vi "SetFieldTCRunner.vi"() -> ()   [LabVIEW 2019]
uses:
  Components/B_Globals.vi
  Components/DeltaRamp_globals.vi
  Components/Global 2.vi
panel:
  out "Numeric":i32
  in  "Settle [s]":dbl=60.0
  in  "Base Name":string="RT_100uA_dir=vir"
  in  "Start":bool
  in  "Directory":path=path "C:/User Data/gy251/2021628 AEN019D"
  in  "T_high":dbl=4.5
  in  "T_low":dbl=2.5
  in  "T_rate":dbl=0.1
  in  "B _rate":dbl=0.2
  in  "Set Fields":dbl[](array[numeric])=[0.0, 0.1, 0.2, 0.3, 0.4, 0.5, 0.6, 0.7, 0.8, 0.9, 1.0, 1.2, 1.4, 1.6, 1.8, 2.0]
  out "Action":string="Starting Measurement"
  out "Output File":path=path "RT_100uA_dir=vir_set=0p00T"
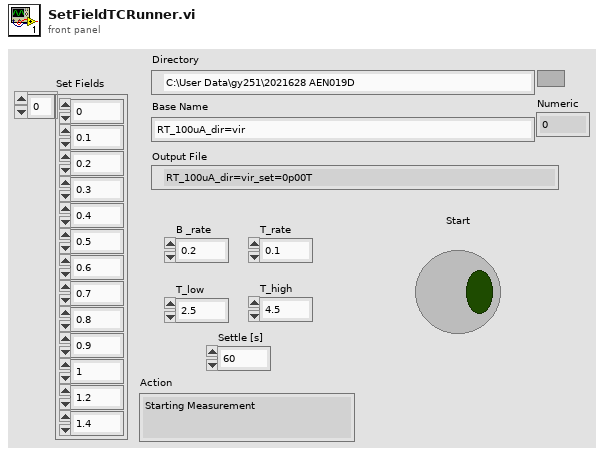
[diagram p1: front panel]
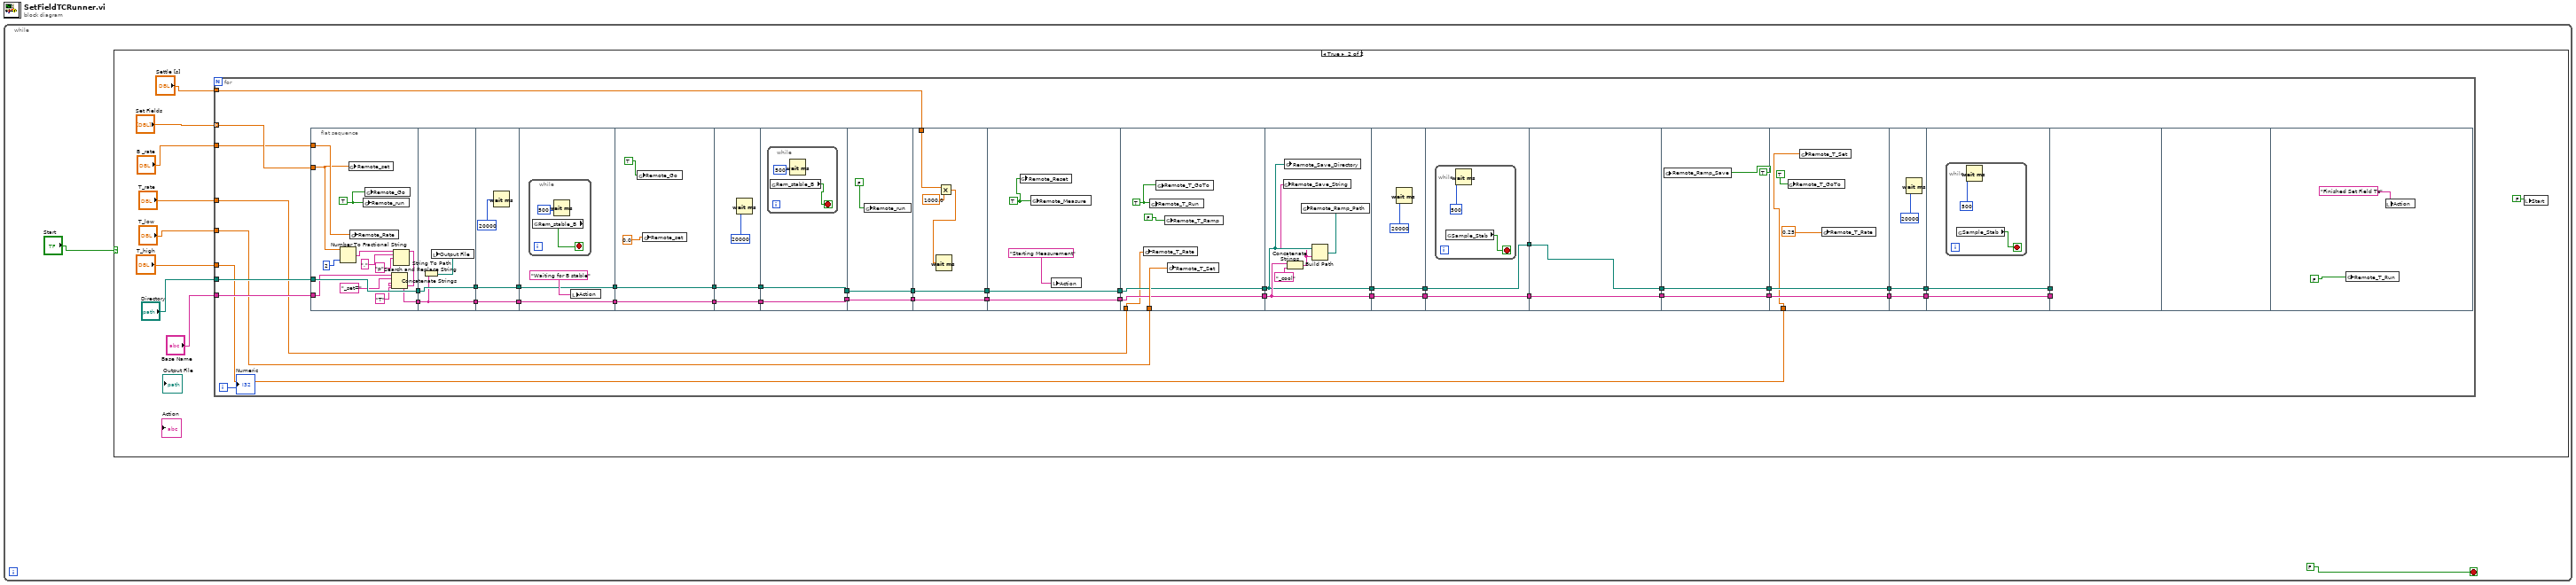
[diagram p0: block diagram]
diagram:
  n1 = while {
    stop <- FALSE stop-if-true
    n2 = case shown="True" "Start" {
      frame False {
      }
      frame True {
        n3 = for {
          tunnel: "Set Fields" -> [w24] mode=indexing
          tunnel: "B _rate" -> [w23]
          tunnel: "Directory" -> [w22]
          tunnel: "Base Name" -> [w21]
          tunnel: "Settle [s]" -> [w20]
          tunnel: "T_low" -> [w19]
          tunnel: "T_rate" -> [w18]
          tunnel: "T_high" -> [w17]
          i -> [w16]
          n4 = flat-sequence {
            tunnel: w24 -> [w66]
            tunnel: w23 -> [w70]
            tunnel: w21 -> [w68]
            tunnel: [w60] -> w58
            tunnel: [w69] -> w57
            tunnel: w22 -> [w69]
            tunnel: [w73] -> w56
            tunnel: w58 -> [w73]
            tunnel: w57 -> [w74]
            tunnel: [w74] -> w55
            tunnel: w56 -> [w77]
            tunnel: [w77] -> w54
            tunnel: w55 -> [w76]
            tunnel: [w76] -> w53
            tunnel: [w79] -> w52
            tunnel: w54 -> [w79]
            tunnel: [w78] -> w51
            tunnel: w53 -> [w78]
            tunnel: [w84] -> w50
            tunnel: w52 -> [w84]
            tunnel: [w83] -> w49
            tunnel: w51 -> [w83]
            tunnel: [w88] -> w48
            tunnel: w50 -> [w88]
            tunnel: [w87] -> w47
            tunnel: w49 -> [w87]
            tunnel: [w91] -> w46
            tunnel: w48 -> [w91]
            tunnel: [w90] -> w45
            tunnel: w47 -> [w90]
            tunnel: w46 -> [w94]
            tunnel: w45 -> [w95]
            tunnel: [w95] -> w44
            tunnel: [w94] -> w43
            tunnel: w20 -> [w100]
            tunnel: [w98] -> w42
            tunnel: w44 -> [w98]
            tunnel: [w97] -> w41
            tunnel: w43 -> [w97]
            tunnel: [w103] -> w40
            tunnel: w42 -> [w103]
            tunnel: [w102] -> w39
            tunnel: w41 -> [w102]
            tunnel: w19 -> [w110]
            tunnel: w40 -> [w107]
            tunnel: w39 -> [w108]
            tunnel: [w108] -> w15
            tunnel: [w107] -> w13
            tunnel: w18 -> [w106]
            tunnel: w15 -> [w116]
            tunnel: [w116] -> w14
            tunnel: w13 -> [w114]
            tunnel: [w114] -> w12
            tunnel: [w118] -> w38
            tunnel: w14 -> [w118]
            tunnel: [w117] -> w37
            tunnel: w12 -> [w117]
            tunnel: w38 -> [w120]
            tunnel: w37 -> [w121]
            tunnel: [w121] -> w36
            tunnel: [w120] -> w35
            tunnel: w36 -> [w124]
            tunnel: w35 -> [w125]
            tunnel: [w124] -> w34
            tunnel: [w125] -> w33
            tunnel: w34 -> [w128]
            tunnel: [w128] -> w32
            tunnel: w33 -> [w127]
            tunnel: [w127] -> w31
            tunnel: w32 -> [w130]
            tunnel: w31 -> [w131]
            tunnel: [w131] -> w30
            tunnel: [w130] -> w29
            tunnel: w17 -> [w129]
            tunnel: [w135] -> w28
            tunnel: w30 -> [w135]
            tunnel: [w134] -> w27
            tunnel: w29 -> [w134]
            tunnel: w28 -> [w138]
            tunnel: [w138] -> w26
            tunnel: [w137] -> w25
            tunnel: w27 -> [w137]
            tunnel: w26 -> [_]
            tunnel: w25 -> [_]
            frame #0 {
              w71 = TRUE
              n5 = Number To Fractional String(number=w66, precision (6)=2) -> (F-format string=w65:string)  [unwired: 2 in]
              n6 = global write "B_Globals.vi" "Remote_set"(w66) -> ()
              n7 = global write "B_Globals.vi" "Remote_Rate"(w70) -> ()
              n8 = global write "B_Globals.vi" "Remote_run"(w71) -> ()
              n9 = global write "B_Globals.vi" "Remote_Go"(w71) -> ()
              n10 = Search and Replace String(input string=w65, search string=".", replace string="p") -> (result string=w62:string)  [unwired: 5 in, 3 out]
              n11 = Concatenate Strings(w68, "_set=", w62, "T") -> (w60:string)
            }
            frame #1 {
              n12 = String To Path(string=w73) -> (path=w72:path)
              n13 = local write "Output File"(w72) -> ()
            }
            frame #2 {
              n14 = Wait (ms)(milliseconds to wait=20000) -> ()  [unwired: 1 out]
            }
            frame #3 {
              n15 = while {
                stop <- w81 stop-if-true
                n16 = global read "B_Globals.vi" "Rem_stable_B"() -> (w81:bool)
                n17 = Wait (ms)(milliseconds to wait=500) -> ()  [unwired: 1 out]
              }
              n18 = local write "Action"("Waiting for B stable") -> ()
            }
            frame #4 {
              n19 = global write "B_Globals.vi" "Remote_Go"(TRUE) -> ()
              n20 = global write "B_Globals.vi" "Remote_set"(0.0) -> ()
            }
            frame #5 {
              n21 = Wait (ms)(milliseconds to wait=20000) -> ()  [unwired: 1 out]
            }
            frame #6 {
              n22 = while {
                stop <- w93 stop-if-true
                n23 = global read "B_Globals.vi" "Rem_stable_B"() -> (w93:bool)
                n24 = Wait (ms)(milliseconds to wait=500) -> ()  [unwired: 1 out]
              }
            }
            frame #7 {
              n25 = global write "B_Globals.vi" "Remote_run"(FALSE) -> ()
            }
            frame #8 {
              n26 = Multiply(x=w100, y=1000.0) -> (x*y=w99:dbl)
              n27 = Wait (ms)(milliseconds to wait=w99) -> ()  [unwired: 1 out]
            }
            frame #9 {
              w105 = TRUE
              n28 = global write "DeltaRamp_globals.vi" "Remote_Reset"(w105) -> ()
              n29 = global write "DeltaRamp_globals.vi" "Remote_Measure"(w105) -> ()
              n30 = local write "Action"("Starting Measurement") -> ()
            }
            frame #10 {
              w111 = TRUE
              n31 = global write "Global 2.vi" "Remote_T_Rate"(w106) -> ()
              n32 = global write "Global 2.vi" "Remote_T_Run"(w111) -> ()
              n33 = global write "Global 2.vi" "Remote_T_GoTo"(w111) -> ()
              n34 = global write "Global 2.vi" "Remote_T_Ramp"(FALSE) -> ()
              n35 = global write "Global 2.vi" "Remote_T_Set"(w110) -> ()
            }
            frame #11 {
              n36 = global write "DeltaRamp_globals.vi" "Remote_Save_Directory"(w114) -> ()
              n37 = Concatenate Strings(w116, "_cool") -> (w113:string)
              n38 = global write "DeltaRamp_globals.vi" "Remote_Save_String"(w113) -> ()
              n39 = Build Path(base path=w114, name or relative path=w113) -> (appended path=w112:path)
              n40 = global write "DeltaRamp_globals.vi" "Remote_Ramp_Path"(w112) -> ()
            }
            frame #12 {
              n41 = Wait (ms)(milliseconds to wait=20000) -> ()  [unwired: 1 out]
            }
            frame #13 {
              n42 = while {
                stop <- w123 stop-if-true
                n43 = global read "Global 2.vi" "Sample_Stab"() -> (w123:bool)
                n44 = Wait (ms)(milliseconds to wait=500) -> ()  [unwired: 1 out]
              }
            }
            frame #14 {
            }
            frame #15 {
              n45 = global write "DeltaRamp_globals.vi" "Remote_Ramp_Save"(TRUE) -> ()
            }
            frame #16 {
              n46 = global write "Global 2.vi" "Remote_T_GoTo"(TRUE) -> ()
              n47 = global write "Global 2.vi" "Remote_T_Set"(w129) -> ()
              n48 = global write "Global 2.vi" "Remote_T_Rate"(0.25) -> ()
            }
            frame #17 {
              n49 = Wait (ms)(milliseconds to wait=20000) -> ()  [unwired: 1 out]
            }
            frame #18 {
              n50 = while {
                stop <- w140 stop-if-true
                n51 = global read "Global 2.vi" "Sample_Stab"() -> (w140:bool)
                n52 = Wait (ms)(milliseconds to wait=500) -> ()  [unwired: 1 out]
              }
            }
            frame #19 {
            }
            frame #20 {
            }
            frame #21 {
              n53 = global write "Global 2.vi" "Remote_T_Run"(FALSE) -> ()
              n54 = local write "Action"("Finished Set Field Tc") -> ()
            }
          }
          "Numeric" <- w16
        }
        n55 = local write "Start"(FALSE) -> ()
      }
    }
  }
